vi "Actor Core.vi"(8 "error in":errorcluster, 11 "Monitor Controller in":refnum<class "Monitor Controller.lvclass">) -> (0 "error out":errorcluster, 3 "Actor out":refnum<class "Actor.lvclass">)   [LabVIEW 2018, in "Monitor Controller.lvclass"]
doc: "(<B>Filename</B>: Actor Framework.lvlib:Actor.lvclass:Actor Core.vi)\n\nReceives messages to the actor, reacts to them, and initiates any error handling that may shut the actor down.\n\nDescendant classes may override this VI to append parallel tasks for the actor to complete while it handles messages. Overrides use the Call Parent Method node."
uses:
  Monitor Controller.lvclass
  <vilib>/ActorFramework/Actor/Actor.lvclass
  Monitor Controller Configuration.ctl
  Process Controller/Process Controller.lvclass
panel:
  in  "Configuration":T1={"Update period"=1.0, "Repeat times"=-1, "Open plot"=TRUE, "File defragment period"=600.0, "Timestamp data points"=FALSE, "Re-plot rate limit"=0.95} {"Re-plot rate limit" format="%#_6ps"; "File defragment period" format="%#_6ps"; "Update period" min=0.01 max=100.0 format="%#_6ps"}
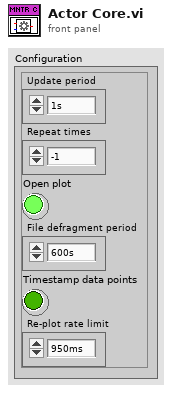
[diagram p1: front panel]
types:
  T1 = typedef "Monitor Controller Configuration.ctl" = cluster{"Update period":dbl, "Repeat times":i32, "Open plot":bool, "File defragment period":dbl, "Timestamp data points":bool, "Re-plot rate limit":dbl}
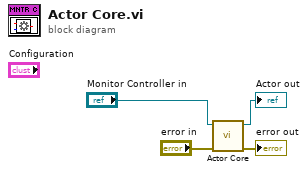
[diagram p0: block diagram]
diagram:
  n1 = call-parent "Actor Core.vi"("error in"="error in", "Measure Object in"="Monitor Controller in") -> ("error out"=→"error out":errorcluster, "Actor out"=→"Actor out":refnum<class "Actor.lvclass">)  [unwired: 8 in]
